vi "Blend Overlay Color with Background.vi"(4 "Overlay Color Value":T1, 6 "Image Scale Factor":sgl, 7 "Blend Overlay with Background":bool, 8 "error in (no error)":errorcluster, 9 "Image Display Range":cluster{"Min Value":sgl, "Max Value":sgl}={"Min Value"=nan, "Max Value"=nan}, 10 "Image Color Array":cluster{"Red":u8, "Green":u8, "Blue":u8}[](array[cluster]), 11 "Pixel Value":sgl) -> (0 "error out":errorcluster, 3 "Scaled/Blended Overlay Color Value":T1)   [LabVIEW 2021, in "Image.lvlib"]
doc: "Computes the scaled or blended pixel's overlay color based on its <B>Pixel Intensity</B>, <B>Image Display Range</B> and <B>Image Scale Factor</B>."
uses:
  Image.lvlib
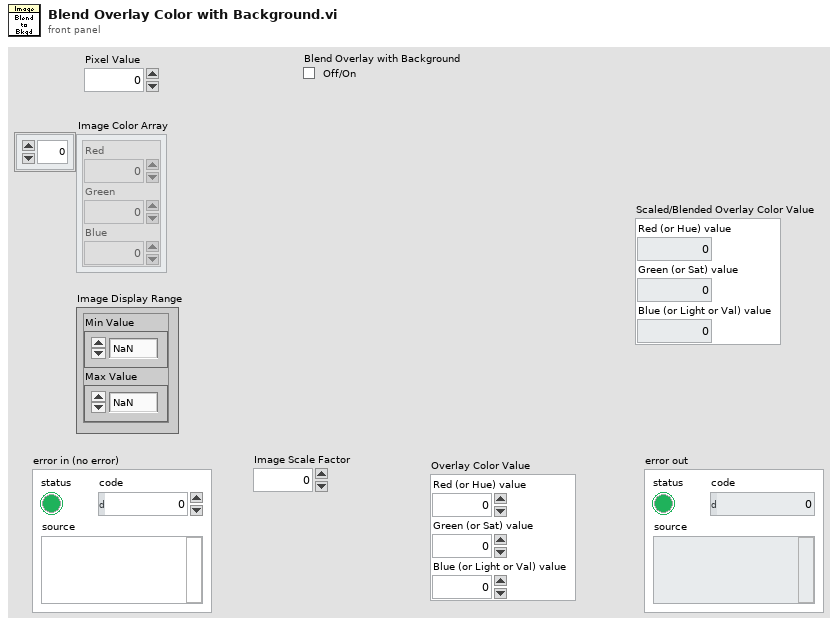
[diagram p1: front panel]
types:
  T1 = cluster{"Red (or Hue) value":u8, "Green (or Sat) value":u8, "Blue (or Light or Val) value":u8}
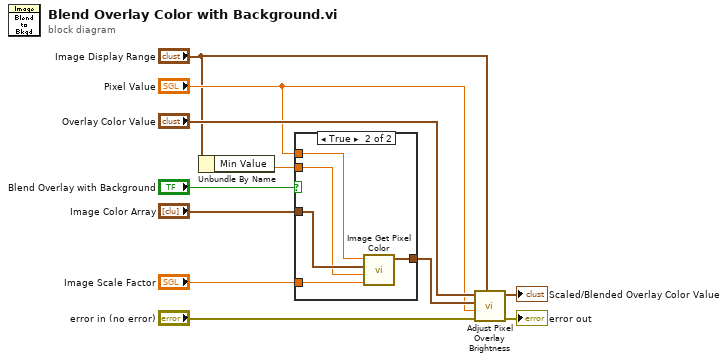
[diagram p0: block diagram]
diagram:
  n1 = Unbundle By Name("Image Display Range") -> ("Min Value"=w1:sgl)
  n2 = case shown="True" "Blend Overlay with Background" {
    tunnel: [_ w16] -> w4
    tunnel: "Image Color Array" -> [_ w15]
    tunnel: w1 -> [_ w14]
    tunnel: "Image Scale Factor" -> [_ w13]
    tunnel: "Pixel Value" -> [_ w12]
    frame False {
    }
    frame True {
      n3 = call "Image Get Pixel Color.vi"("Image Scale Factor (256 colors)"=w13, "Image Range Min Value"=w14, "1D Color Array"=w15, "Image Pixel Value"=w12) -> ("Pixel Color (black)"=w16:T1)  [unwired: 7 in]
    }
  }
  n4 = call "Adjust Pixel Overlay Brightness.vi"("Image Display Range"="Image Display Range", "Error In"="error in (no error)", "Pixel Intensity"="Pixel Value", "Pixel Color Value"=w4, "Overlay Color Value"="Overlay Color Value") -> ("Error Out"=→"error out":errorcluster, "Overlay Color Value"=→"Scaled/Blended Overlay Color Value":T1)  [unwired: 5 in]
